vi "Concatenate2.vi"(2 "b":refnum<class "Bytestream.lvclass">, 3 "a":refnum<class "Bytestream.lvclass">) -> (0 "d":refnum<class "Bytestream.lvclass">, 1 "c":refnum<class "Bytestream.lvclass">)   [LabVIEW 2020, in "NI_Bytestream.lvlib" / "Bytestream.lvclass"]
uses:
  <vilib>/Array/Bytestream/Bytestream.lvclass
  <vilib>/Array/Bytestream/Bytestream.lvclass/Bytestream.ctl
  <vilib>/Array/Bytestream/Count Allocated Datums.vi
  <vilib>/Array/Bytestream/Count Datums.vi
  <vilib>/Array/Bytestream/Get Logical Datum.vi
  <vilib>/Array/Bytestream/Datum Size.vi
  <vilib>/Array/Bytestream/Grow Datum Array.vi
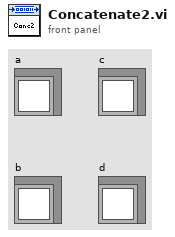
[diagram p1: front panel]
types:
  T1 = typedef "NI_Bytestream.lvlib/Bytestream.lvclass/Datum.ctl" = cluster{"array":u8[], "index":i32}
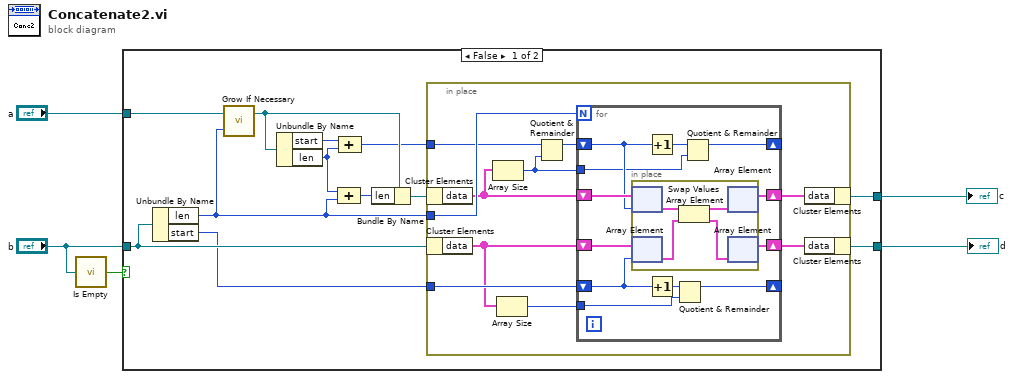
[diagram p0: block diagram]
diagram:
  n1 = call <vilib>:"Is Empty.vi"("a"="b") -> ("empty?"=w1:bool)
  n2 = case shown="False" w1 {
    tunnel: [w15 w45] -> w4
    tunnel: "a" -> [w17 w45]
    tunnel: "b" -> [w16 w44]
    tunnel: [w7 w44] -> w2
    frame False {
      n3 = Unbundle By Name(w16) -> ("len"=w10:i32, "start"=w11:i32)
      n4 = call <vilib>:"Grow If Necessary.vi"("number of additional datums (1)"=w10, "bytestream in"=w17) -> ("bytestream out"=w14:refnum<class "Bytestream.lvclass">)  [unwired: 1 in]
      n5 = Unbundle By Name(w14) -> ("start"=w9:i32, "len"=w8:i32)
      n6 = Compound Arithmetic op=ADD(w8, w10) -> (w13:i32)
      n7 = Compound Arithmetic op=ADD(w9, w8) -> (w6:i32)
      n8 = Bundle By Name(cluster=w14, "len"=w13) -> (w12:refnum<class "Bytestream.lvclass">)
      n9 = in-place {
        in-place-border: w11 -> [w26]
        in-place-border: w10 -> [w27]
        in-place-border: w6 -> [w20]
        n10 = in-place-cluster #1(w12) -> ("data"=w23:T1[])
        n11 = in-place-cluster #2(w16) -> ("data"=w22:T1[])
        n12 = Array Size(array=w23) -> (size(s)=w19:i32)
        n13 = Array Size(array=w22) -> (size(s)=w21:i32)
        n14 = Quotient & Remainder(x=w20, y=w19) -> (x-y*floor(x/y)=w18:i32)  [unwired: 1 out]
        n15 = for {
          N: w27 -> [_]
          shift-right: [w30] -> _
          shift-left: w18 -> [w35]
          shift-right: [w32] -> _
          shift-left: w26 -> [w34]
          shift-right: [w37] -> w25
          shift-left: w23 -> [w39]
          shift-right: [w36] -> w24
          shift-left: w22 -> [w38]
          tunnel: w19 -> [w29]
          tunnel: w21 -> [w28]
          n16 = in-place {
            n17 = in-place-array #3(w39, w35) -> (w43:T1)
            n18 = in-place-array #4(w38, w34) -> (w42:T1)
            n19 = Swap Values(12:w43, 14:w42) -> (1:w41:T1, 3:w40:T1)  [unwired: 1 in]
            n20 = in-place-array #3(w41) -> (w37:T1[])  [unwired: 1 out]
            n21 = in-place-array #4(w40) -> (w36:T1[])  [unwired: 1 out]
          }
          n22 = Increment(x=w35) -> (x+1=w31:i32)
          n23 = Increment(x=w34) -> (x+1=w33:i32)
          n24 = Quotient & Remainder(x=w33, y=w28) -> (x-y*floor(x/y)=w32:i32)  [unwired: 1 out]
          n25 = Quotient & Remainder(x=w31, y=w29) -> (x-y*floor(x/y)=w30:i32)  [unwired: 1 out]
        }
        n26 = in-place-cluster #1("data"=w25) -> (w15:refnum<class "Bytestream.lvclass">)
        n27 = in-place-cluster #2("data"=w24) -> (w7:refnum<class "Bytestream.lvclass">)
      }
    }
    frame True {
    }
  }
  "c" <- w4
  "d" <- w2
